vi "pulse from memory 1spc_v3.vi"(7 "stop this pulse":bool, 8 "run":bool=TRUE, 9 "referenses":T4={"clock x2"="IO Socket\\Data Clock 2x", "Memory In"="pulse on memory"}, 10 "start this pulse":bool, 11 "PDW":T2={"PW"=0, "frequency shift"=0.0, "amp"=0.9999923706054688, "mode type"=enum."CW", "mode depth"=0, "mode filter"=0, "phase shift"=0.0, "pulse shape filter"=0} {"frequency shift" format="%#_12f"}) -> (1 "free DDS":bool, 2 "output valid":bool=TRUE, 3 "IQ out":T1)   [LabVIEW 2021]
uses:
  pulse_tx_vis/pdw.ctl
  pulse_tx_vis/CTL/mode_type.ctl
  <instrlib>/_niInstr/DSP/v1/Shared/Public/IQ Data.ctl
  <instrlib>/_niInstr/DSP/v1/FPGA/Public/Sub VIs/Data Conversion/U32 to IQ - 1 spc - S18.1.vi
  <instrlib>/FlexRIO/API/UsrFpgaDsp/v1/FPGA/HbInt/UsrFpgaDspHbIntIQ_8Cps_1xOC_BWper2_96dB.vi
  <instrlib>/FlexRIO/API/UsrFpgaDsp/v1/FPGA/HbInt/UsrFpgaDspHbIntIQ_4Cps_1xOC_BWper2_89dB.vi
  <instrlib>/FlexRIO/API/UsrFpgaDsp/v1/FPGA/HbInt/UsrFpgaDspHbIntIQ_2Cps_1xOC_BWper2_89dB.vi
  <instrlib>/_niInstr/DSP/v1/FPGA/Public/Sub VIs/Frequency Shift/Frequency Shift - 1 spc.vi
  <vilib>/rvi/DataTransferAndStorage/Container/Common/niFpgaContainerExecOnDevCompGetState.vi
  <vilib>/rvi/Emulation/niFpgaEmulationIsFPGAContextNoSignature.vi
  <vilib>/rvi/DataTransferAndStorage/Container/Common/niFpgaContainerGetUniqueNameForEmu.vi
  <vilib>/rvi/Emulation/niFpgaProcessEmulError.vi
  <vilib>/rvi/Emulation/niFpgaSctlEmulationGetInTimedLoop.vi
  <vilib>/rvi/errors/nirviReportUnexpectedCaseInternalError (U32).vi
  <vilib>/rvi/Memory/Memory_Emulation/niFpgaMemoryEmulationCacheClearOnFirstRun.vi
  <vilib>/rvi/Memory/Memory_Emulation/nirvimemoryEmulationManagerCache_MakeExclusive.vi
  <vilib>/rvi/Memory/Memory_Emulation/niFpgaMemoryEmulationValidateCache.vi
  <vilib>/rvi/Memory/Memory_Emulation/nirvimemoryEmulationManagerCache_InsertValue.vi
  <vilib>/Utility/error.llb/Clear Errors.vi
  <vilib>/rvi/Memory/Memory_Emulation/nirvimemoryEmulationManagerCache_ReleaseExclusive.vi
  <vilib>/rvi/Memory/Memory_Emulation/nirvimemoryEmulationManagerCache_GetValue.vi
  <vilib>/rvi/Memory/Memory_Emulation/nirvimemoryEmulationManagerCache_SetValue.vi
  <vilib>/rvi/Emulation/niFpgaSctlEmulationResourceMgr.vi
  <instrlib>/_niInstr/Basic Elements/v1/FPGA/Private/Count Up U32.vi
  <instrlib>/_niInstr/Basic Elements/v1/FPGA/Private/Count Up U16.vi
  <vilib>/rvi/DataTransferAndStorage/Container/XNode/niFpgaContainer.xnode
  <vilib>/rvi/Memory/Memory_Emulation/niFpgaMemoryEmulationRefIn.vi
  <instrlib>/_niInstr/DSP/v1/Shared/niInstr DSP v1 Shared.lvlib
  <instrlib>/_niInstr/DSP/v1/FPGA/niInstr DSP v1 FPGA.lvlib
  <instrlib>/_niInstr/Basic Elements/v1/FPGA/niInstr Basic Elements v1 FPGA.lvlib
  <instrlib>/FlexRIO/API/UsrFpgaDsp/v1/FPGA/HbInt/UsrFpgaDsp HbInt v1 FPGA.lvlib
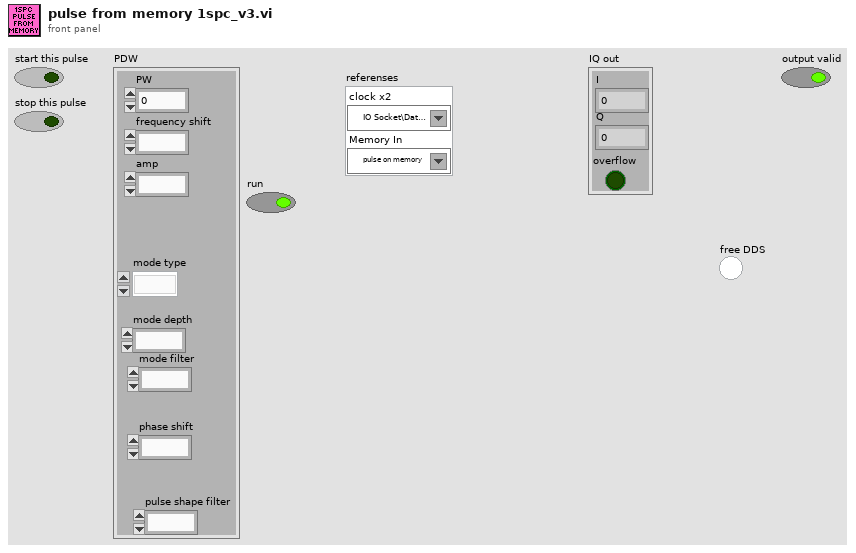
[diagram p1: front panel]
types:
  T1 = typedef "niInstr DSP v1 Shared.lvlib/IQ Data.ctl" = cluster{"I":fxp<+/-,18,1>, "Q":fxp<+/-,18,1>, "overflow":bool}
  T2 = typedef "pdw.ctl" = cluster{"PW":u32, "frequency shift":fxp<+/-,48,0>, "amp":fxp<+/-,18,1>, "mode type":T3, "mode depth":u32, "mode filter":u8, "phase shift":fxp<+/-,16,1>, "pulse shape filter":u8}
  T3 = typedef "mode_type.ctl" = enum8{"CW", "from memory 1", "NC - cw", "LFM", "BPSK", "QPSK"}
  T4 = cluster{"clock x2":refnum<k21>, "Memory In":refnum<k21>}
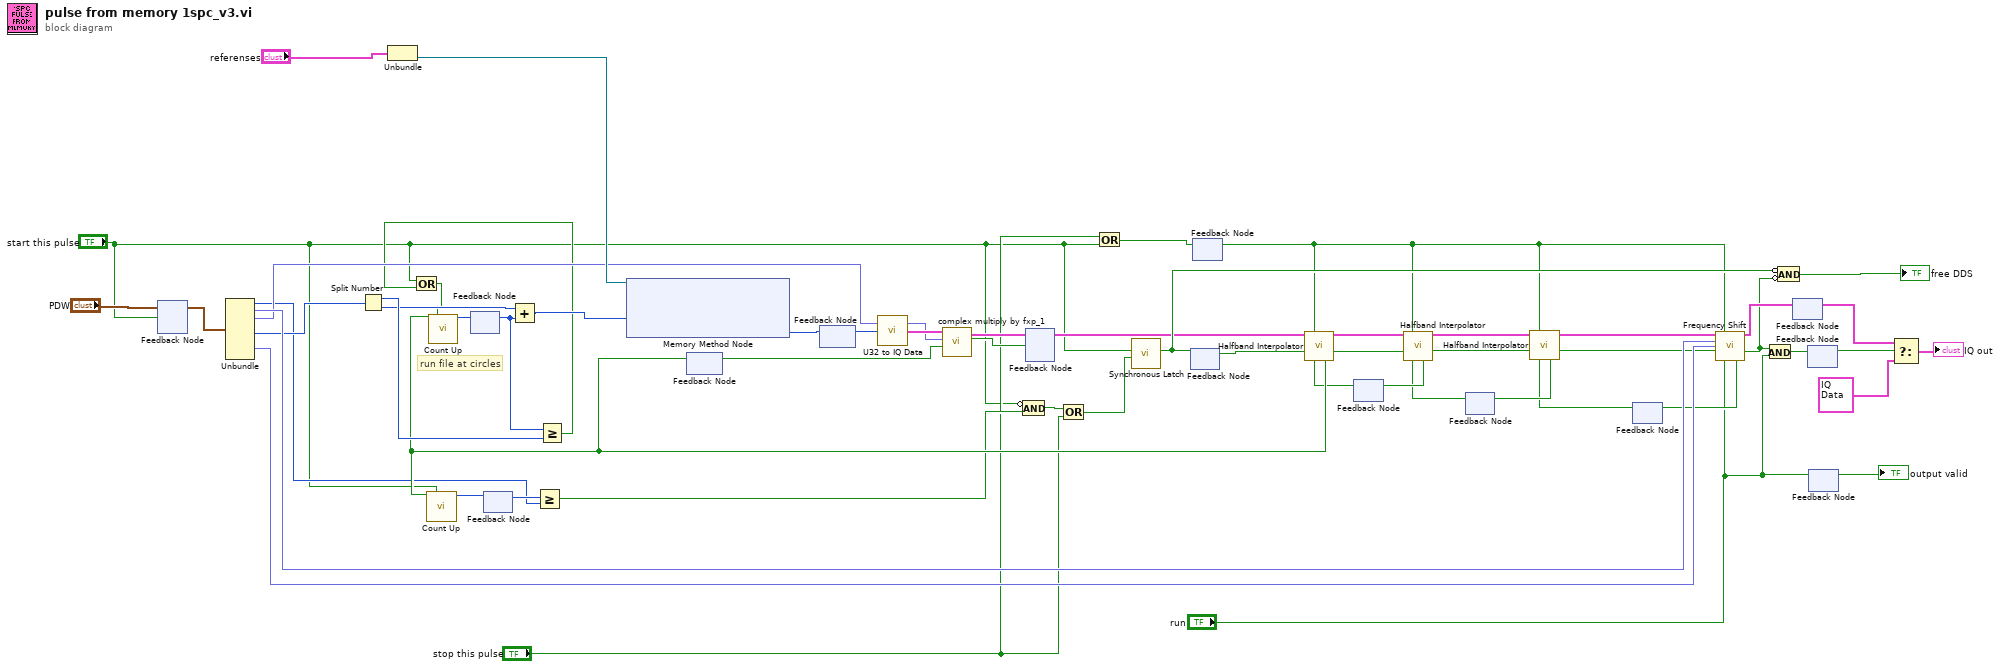
[diagram p0: block diagram]
diagram:
  # "run file at circles"
  n1 = feedback #1() -> (w50:T2)  [unwired: 1 in]
  n2 = feedback-in #1("PDW", "start this pulse") -> ()
  n3 = Unbundle(w50) -> ("PW"=w22:u32, "frequency shift"=w55:fxp<+/-,48,0>, "amp"=w44:fxp<+/-,18,1>, "mode depth"=w28:u32, "phase shift"=w54:fxp<+/-,16,1>)  [unwired: 3 out]
  n4 = Split Number(x=w28) -> (hi(x)=w49:u16, lo(x)=w43:u16)
  n5 = Unbundle("referenses") -> ("Memory In"=w52:refnum<k21>)  [unwired: 1 out]
  n6 = feedback #2() -> (w41:u16)  [unwired: 1 in]
  n7 = feedback #3() -> (w23:u32)  [unwired: 1 in]
  n8 = Add(x=w43, y=w41) -> (x+y=w40:u16)
  n9 = Greater Or Equal?(x=w23, y=w22) -> (x >= y?=w21:bool)
  n10 = Greater Or Equal?(x=w41, y=w49) -> (x >= y?=w25:bool)
  n11 = Or(x="start this pulse", y=w25) -> (x .or. y?=w26:bool)
  n12 = xnode ("Memory Method Node")("Address"=w40, "Memory In"=w52) -> ("Data"=w57:u32)  [unwired: 1 out]
  n13 = feedback #4() -> (w45:bool)  [unwired: 1 in]
  n14 = feedback #5() -> (w56:u32)  [unwired: 1 in]
  n15 = feedback-in #5(w57) -> ()
  n16 = call-poly <instrlib>:"U32 to IQ Data.vi"("U32 data"=w56) -> ("IQ data"=w47:T1)  [unwired: 14 in]
  n17 = call "complex multiply by fxp_1.vi"("input valid"=w45, "amp"=w44, "IQ data"=w47) -> ("data valid"=w48:bool, "output cluster"=w46:T1)  [unwired: 7 in]
  n18 = Compound Arithmetic op=AND(invert "start this pulse", w21) -> (w5:bool)
  n19 = feedback #6() -> (w30:T1)  [unwired: 1 in]
  n20 = feedback-in #6(w46, w48) -> ()
  n21 = Or(x=w5, y="stop this pulse") -> (x .or. y?=w1:bool)
  n22 = Or(x="stop this pulse", y="start this pulse") -> (x .or. y?=w2:bool)
  n23 = call <instrlib>:"Synchronous Latch.vi"("clear"=w1, "set"="start this pulse") -> ("out"=w35:bool)  [unwired: 9 in]
  n24 = feedback #7() -> (w29:bool)  [unwired: 1 in]
  n25 = feedback-in #7(w35) -> ()
  n26 = feedback #8() -> (w20:bool)  [unwired: 1 in]
  n27 = feedback-in #8(w2) -> ()
  n28 = feedback #9() -> (w18:bool)  [unwired: 1 in]
  n29 = call-poly "Halfband Interpolator.vi"("data in"=w30, "reset"=w20, "input valid"=w29, "ready for output (T)"=w18) -> ("data out"=w34:T1, "output valid"=w31:bool, "ready for input"=w24:bool)  [unwired: 9 in]
  n30 = call-poly <instrlib>:"Count Up.vi"("increment"=w24, "reset"="start this pulse") -> ("count out"=w27:u32)  [unwired: 13 in]
  n31 = call-poly <instrlib>:"Count Up.vi"("increment"=w24, "reset"=w26) -> ("count out"=w42:u16)  [unwired: 13 in]
  n32 = feedback-in #2(w42) -> ()
  n33 = feedback-in #3(w27) -> ()
  n34 = feedback-in #4(w24) -> ()
  n35 = feedback #10() -> (w16:bool)  [unwired: 1 in]
  n36 = call-poly "Halfband Interpolator.vi"("data in"=w34, "reset"=w20, "input valid"=w31, "ready for output (T)"=w16) -> ("data out"=w33:T1, "output valid"=w32:bool, "ready for input"=w19:bool)  [unwired: 9 in]
  n37 = feedback-in #9(w19) -> ()
  n38 = feedback #11() -> (w10:bool)  [unwired: 1 in]
  n39 = call-poly "Halfband Interpolator.vi"("data in"=w33, "reset"=w20, "input valid"=w32, "ready for output (T)"=w10) -> ("data out"=w8:T1, "output valid"=w9:bool, "ready for input"=w17:bool)  [unwired: 9 in]
  n40 = feedback-in #10(w17) -> ()
  n41 = call-poly <instrlib>:"Frequency Shift.vi"("data in"=w8, "reset"=w20, "frequency shift"=w55, "phase"=w54, "input valid"=w9, "ready for output (T)"="run") -> ("data out"=w39:T1, "output valid"=w13:bool, "ready for input"=w15:bool)  [unwired: 6 in, 1 out]
  n42 = feedback-in #11(w15) -> ()
  n43 = And(x=w13, y="run") -> (x .and. y?=w12:bool)
  n44 = Compound Arithmetic op=AND(invert w35, invert w13) -> (→"free DDS":bool)
  n45 = feedback #12() -> (w38:T1)  [unwired: 1 in]
  n46 = feedback-in #12(w39) -> ()
  n47 = feedback #13() -> (w37:bool)  [unwired: 1 in]
  n48 = feedback-in #13(w12) -> ()
  n49 = feedback #14() -> (→"output valid":bool)  [unwired: 1 in]
  n50 = feedback-in #14("run") -> ()
  n51 = Select(t=w38, s=w37, f=T1 {"I"=0.0, "Q"=0.0, "overflow"=FALSE} ("data")) -> (s? t:f=→"IQ out":T1)
